vi "Robot Global Data.vi"() -> ()   [LabVIEW 2016]
doc: "This global VI can contain as many global variables as you need. Place a control on the panel, give it a good name. To read or write to it from a VI, drag the icon to the diagram of that VI. You can also drag from the project. Click on the node to change which global you access. You shouldn't have multiple locations writing to a global or it will cause a race-condition."
uses:
  <vilib>/Rock Robotics/WPI/Camera/WPI_CameraImageSize.ctl
  <vilib>/Rock Robotics/WPI/DriverStation/WPI_DriverStationRobotMode2.ctl
panel:
  in  "shooter velocity":dbl=-1080.0
  out "boiler size y (1-200) 2":dbl
  out "boiler size x (1-320) 2":dbl
  out "boiler y (0-119) 2":dbl
  out "boiler center x (0-319) 2":dbl
  out "boiler pixy status":dbl
  in  "Shooter Serial Name":refnum<visa-resource-name>="ASRL3::INSTR"
  out "Navx auto starting position":dbl
  out "Right Velocity":dbl
  out "Left Velocity":dbl
  out "Zero Sensor":bool
  out "Aiming Encoder Offset":dbl
  out "Shooter Encoder Offset":dbl
  out "Aiming Encoder":dbl
  out "Shooter Encoder":dbl
  in  "Right Encoder Offset":dbl
  in  "Left Encoder Offset":dbl
  out "Left Encoder":dbl
  out "Right Encoder":dbl
  out "Navx fused heading":dbl
  out "size y (1-200)":dbl
  out "size x (1-320)":dbl
  out "center y (0-119)":dbl
  out "center x (0-319)":dbl
  out "status":dbl
  in  "Gear peg Serial Name":refnum<visa-resource-name>="ASRL3::INSTR"
  in  "USB In":string
  in  "Robot Mode":T1
  in  "image size":T2=enum."320x240"
  in  "Enable Vision":bool
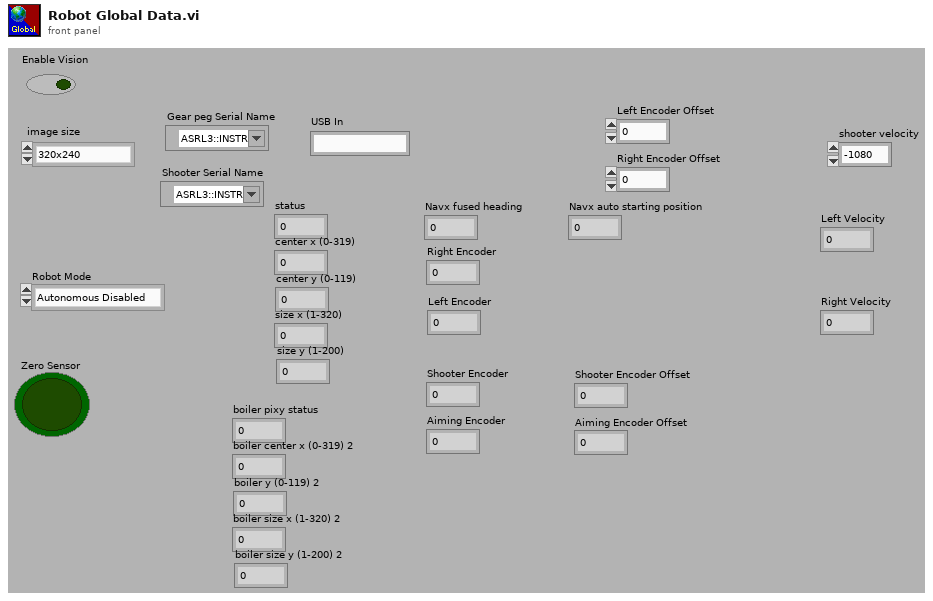
[diagram p1: front panel]
types:
  T1 = typedef "WPI_DriverStationRobotMode2.ctl" = enum16{"Autonomous Disabled", "Autonomous Enabled", "Teleop Disabled", "Teleop Enabled", "Disconnected", "Finish", "Test Disabled", "Test Enabled", "Emergency Stopped"}
  T2 = typedef "WPI_CameraImageSize.ctl" = enum16{"640x480", "320x240", "160x120", "Custom"}
diagram:
